vi "UTIL Progress Bar Get Abort.vi"(8 "error in (no error)":errorcluster, 11 "reference in":refnum<vi>) -> (0 "error out":errorcluster, 2 "Abort":bool, 3 "reference out":refnum<vi>)   [LabVIEW 2019]
doc: "10/01/2010\n\nNational Analytics (TLE)\n\nRead the status of the Abort button."
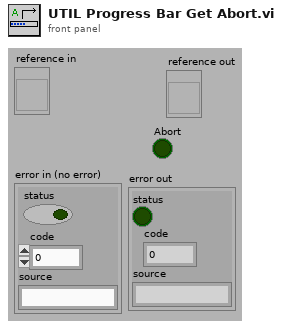
[diagram p1: front panel]
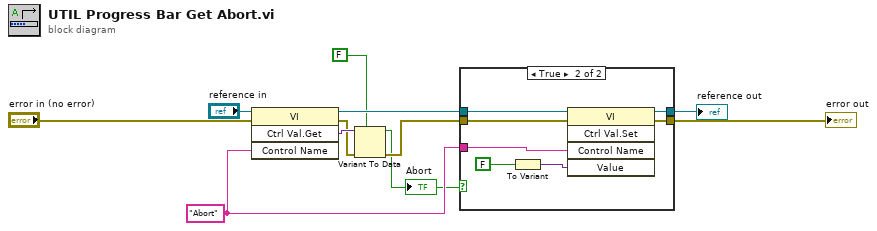
[diagram p0: block diagram]
diagram:
  w9 = "Abort" ("Control Name")
  n1 = invoke class="VI" method="Ctrl Val.Get"(reference="reference in", error in="error in (no error)", "Control Name"=w9) -> (reference out=w8:refnum<vi>, error out=w3:errorcluster, "Get Control Value Variant"=w5:variant)  [unwired: 1 in, 1 out]
  n2 = Variant To Data(error in=w3, type=FALSE ("Abort"), Variant=w5) -> (data=w1:bool, error out=w2:errorcluster)
  "Abort" <- w1
  n3 = case shown="True" w1 {
    tunnel: w9 -> [_ w20]
    tunnel: w2 -> [w12 w19]
    tunnel: w8 -> [w13 w18]
    tunnel: [w13 w17] -> w7
    tunnel: [w12 w16] -> w6
    frame False {
    }
    frame True {
      n4 = To Variant(anything=FALSE ("Abort")) -> (Variant=w14:variant)
      n5 = invoke class="VI" method="Ctrl Val.Set"(reference=w18, error in=w19, "Control Name"=w20, "Value"=w14) -> (reference out=w17:refnum<vi>, error out=w16:errorcluster)  [unwired: 1 in, 3 out]
    }
  }
  "reference out" <- w7
  "error out" <- w6
